vi "RefreshThermSettingUI.vi"(3 "Thermocouple":refnum<vi>) -> ()   [LabVIEW 2024]
uses:
  <vilib>/regexp/Match Regular Expression.xnode
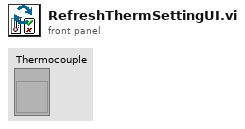
[diagram p1: front panel]
types:
  T1 = enum8{"Enabled", "Disabled", "Disabled and Grayed Out"}
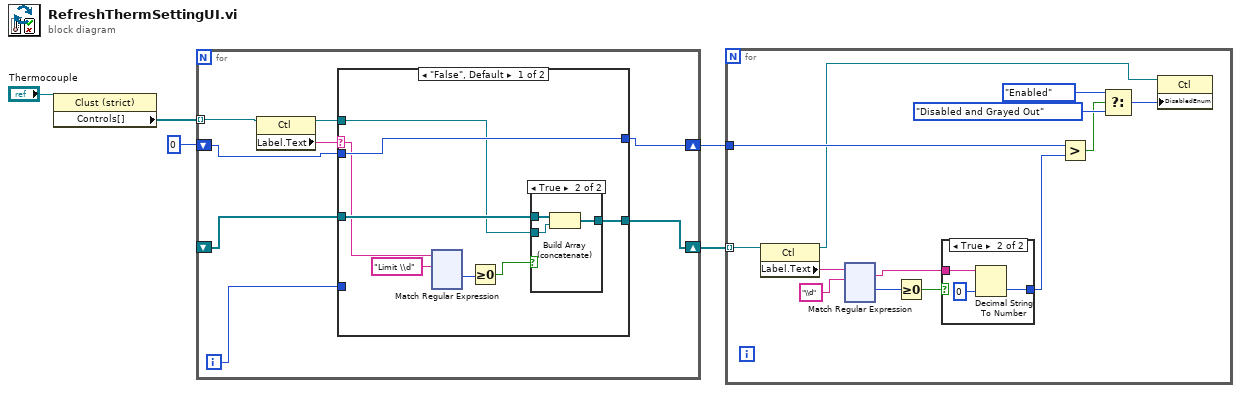
[diagram p0: block diagram]
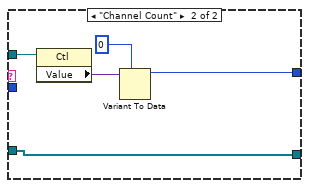
[diagram p4: hidden frame]
diagram:
  n1 = property class="Clust (strict)"(reference="Thermocouple") -> ("Controls[]"=w4:refnum<vi>[])  [unwired: 1 in, 2 out]
  n2 = for {
    tunnel: w4 -> [w13] mode=indexing
    shift-right: [w10] -> w1
    shift-left: 0 -> [w9]
    shift-right: [w6] -> w2
    shift-left: _ -> [w7]
    i -> [w8]
    n3 = property class="Ctl"(reference=w13) -> (reference out=w11:refnum<vi>, "Label.Text"=w12:string)  [unwired: 1 in, 1 out]
    n4 = case shown="\"False\", Default" w12 {
      selector: w12 -> [w17 _]
      tunnel: w11 -> [w19 w147]
      tunnel: [w21 w144] -> w10
      tunnel: w9 -> [w21 _]
      tunnel: w8 -> [_ _]
      tunnel: w7 -> [w20 w143]
      tunnel: [w18 w143] -> w6
      frame "False", Default {
        n5 = xnode "Match Regular Expression"("input string"=w17, "regular expression"="Limit \\d") -> ("offset past match"=w15:i32)  [unwired: 4 in, 4 out]
        n6 = Greater Or Equal To 0?(x=w15) -> (x >= 0?=w14:bool)
        n7 = case shown="True" w14 {
          tunnel: w20 -> [w139 w142]
          tunnel: w19 -> [_ w141]
          tunnel: [w139 w140] -> w18
          frame False {
          }
          frame True {
            n8 = Build Array (concatenate)(w142, w141) -> (w140:refnum<vi>[])
          }
        }
      }
      frame "Channel Count" {
        n9 = property class="Ctl"(reference=w147) -> ("Value"=w146:variant)  [unwired: 1 in, 2 out]
        n10 = Variant To Data(type=0, Variant=w146) -> (data=w144:i32)  [unwired: 1 in, 1 out]
      }
    }
  }
  n11 = for {
    tunnel: w2 -> [w157] mode=indexing
    tunnel: w1 -> [w151]
    n12 = property class="Ctl"(reference=w157) -> (reference out=w148:refnum<vi>, "Label.Text"=w156:string)  [unwired: 1 in, 1 out]
    n13 = xnode "Match Regular Expression"("input string"=w156, "regular expression"="\\d") -> ("whole match"=w152:string, "offset past match"=w154:i32)  [unwired: 4 in, 3 out]
    n14 = Greater Or Equal To 0?(x=w154) -> (x >= 0?=w153:bool)
    n15 = case shown="True" w153 {
      tunnel: w152 -> [_ w163]
      tunnel: [_ w161] -> w150
      frame False {
      }
      frame True {
        n16 = Decimal String To Number(string=w163, default (0L)=0 ("default (0 I32)")) -> (number=w161:i32)  [unwired: 1 in, 1 out]
      }
    }
    n17 = Greater?(x=w151, y=w150) -> (0:w149:bool)
    n18 = Select(t=T1."Enabled" ("Disabled"), s=w149, f=T1."Disabled and Grayed Out" ("Disabled")) -> (s? t:f=w158:T1)
    n19 = property class="Ctl"(reference=w148, "DisabledEnum"=w158) -> ()  [unwired: 1 in, 2 out]
  }
